vi "Tuning.vi"() -> ()   [LabVIEW 2016, in "EV3Group10.lvrbt"]
uses:
  EV3Group10.lvrbt
  <vilib>/NXT/Block Support/NXT_InputPort.ctl
  <vilib>/NXT/Block Support/NXT_OutputPort.ctl
  <vilib>/NXT/Dual Mode Library/Sensors/EV3_Ultrasonic_CM.vi
  <vilib>/NXT/NXTIO Xnodes/NXTIONodeSubVIs/NXTMoveMotors.vi
  <vilib>/NXT/Subs/LVHSConnector.ctl
  <vilib>/NXT/NXTIO Xnodes/AddressXNode/NXTIOAddress.xnode
  <vilib>/NXT/NXTIO Xnodes/NXTIOXNode/NXTIO.xnode
  <vilib>/NXT/LegoClasses/BrickReference/BrickReference.lvclass
panel:
  in  "Stopp":bool
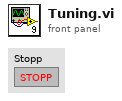
[diagram p1: front panel]
types:
  T1 = typedef "NXT_OutputPort.ctl" = u8
  T2 = typedef "NXT_InputPort.ctl" = u32
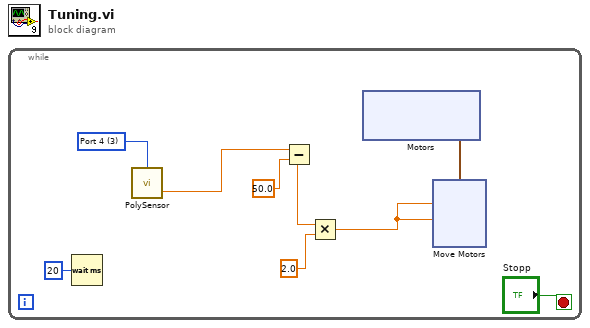
[diagram p0: block diagram]
diagram:
  n1 = while {
    stop <- "Stopp" stop-if-true
    w7 = T2 3 items=["Port 1", "Port 2", "Port 3", "Port 4"] ("Port (Port 1)")
    n2 = Wait (ms)(milliseconds to wait=u32 20 ("Zu wartende ms")) -> ()  [unwired: 1 out]
    n3 = call-poly <vilib>:"PolySensor.vi"("Port (Port 1)"=w7) -> ("Centimeters"=w6:sgl)  [unwired: 2 in, 1 out]
    n4 = Subtract(x=w6, y=50.0) -> (x-y=w5:dbl)
    n5 = Multiply(x=w5, y=2.0) -> (x*y=w3:dbl)
    n6 = xnode "Motors"() -> ("Motor"=w4:cluster{"Port":T1, "Port":T1})
    n7 = xnode "Move Motors"("Power/Speed 2"=w3, "Power/Speed 1"=w3, "Motors"=w4) -> ()  [unwired: 1 in, 1 out]
  }
